vi "ISEG_HVBoardGUI.constructor.vi"(0 "name":string, 2 "data in":string, 5 "error in (no error)":errorcluster) -> (14 "i ref out":refnum<vi>, 16 "data out":string, 19 "error out":errorcluster)   [LabVIEW 2014, in "ISEG_HVBoardGUI.lvlib"]
doc: "This is the constructor of a class.\n\nLicense Agreement for this software:\n\nCopyright (C)\nGesellschaft für Schwerionenforschung, GSI\nPlanckstr. 1\n64291 Darmstadt\nGermany\n\nContact: D.Beck@gsi.de \n\nThis program is free software; you can redistribute it and/or modify it under the terms of the \nGNU General Public License as published by the Free Software Foundation; either version 2 of \nthe license, or (at your option) any later version.\n\nThis program is distributed in the hope that it will be useful, but WITHOUT ANY WARRANTY; \nwithout even the implied warranty of MERCHANTABILITY or FITNESS FOR A PARTICULAR PURPOSE. See the GNU General License for more details (http://www.gnu.org).\n\nGesellschaft für Schwerionenforschung, GSI\nPlanckstr. 1, 64291 Darmstadt, Germany\nFor all questions and ideas contact: M.Richter@gsi.de, H.Brand@gsi.de or D.Beck@gsi.de.\nLast update: 16-JUN-2004"
uses:
  ISEG_HVBoardGUI.lvlib
  ISEG_HVBoardGUI.i attribute.ctl
  CS_Core/CSObj/CSObj.lvlib
  CS_Core/BaseGUI/BaseGUI.lvlib
  CS_Core/CSSystem/CSSystemLib/CSSystemLib.lvlib
panel:
  in  "CLASS.i attribute":T1
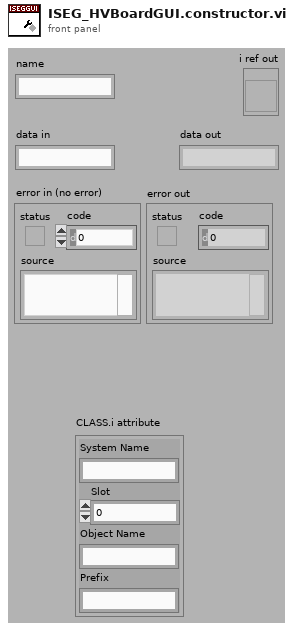
[diagram p1: front panel]
types:
  T1 = typedef "ISEG_HVBoardGUI.lvlib/ISEG_HVBoardGUI.i attribute.ctl" = cluster{"System Name":string, "Slot":i16, "Object Name":string, "Prefix":string}
  T2 = enum16{"SetAttribute", "GetAttribute", "CreateAttribute", "DestroyAttribute", "DestroyAllAtributes"}
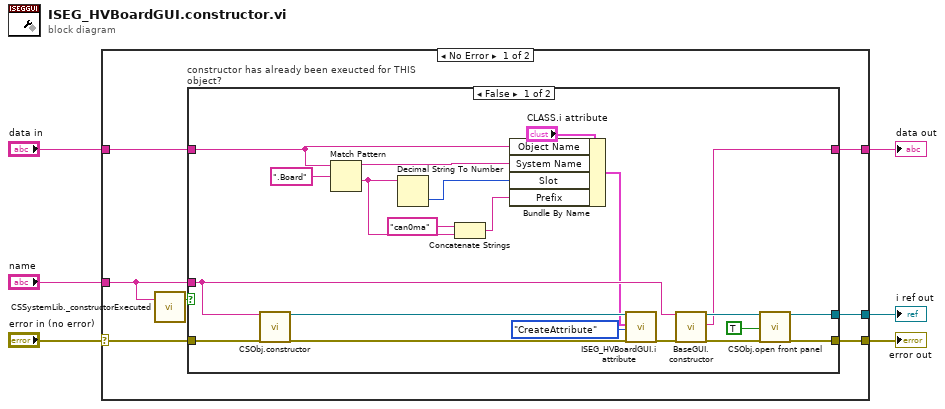
[diagram p0: block diagram]
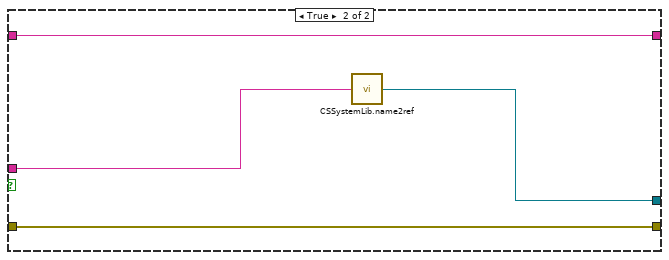
[diagram p2: hidden frame]
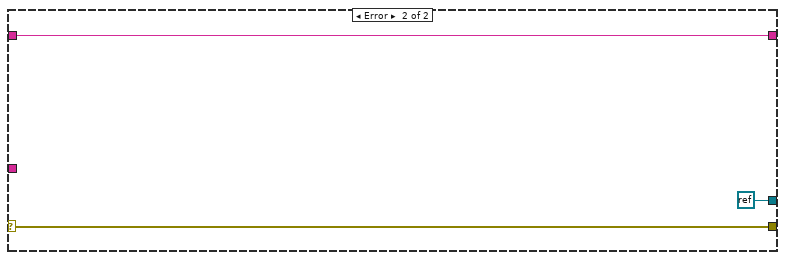
[diagram p3: hidden frame]
diagram:
  n1 = case shown="No Error" "error in (no error)" {
    selector: "error in (no error)" -> [w10 w40]
    tunnel: "data in" -> [w13 w39]
    tunnel: "name" -> [w9 _]
    tunnel: [w12 refnum<k0> refnum] -> w4
    tunnel: [w11 w40] -> w3
    tunnel: [w7 w39] -> w1
    frame No Error {
      n2 = call "CSSystemLib._constructorExecuted.vi"("name"=w9) -> ("constructor executed?"=w8:bool)  [unwired: 18 in]
      n3 = case "constructor has already been exeucted for THIS object?" shown="False" w8 {
        tunnel: w13 -> [w15 w35]
        tunnel: w9 -> [w31 w38]
        tunnel: [w24 w37] -> w12
        tunnel: [w26 w36] -> w11
        tunnel: w10 -> [w29 w36]
        tunnel: [w16 w35] -> w7
        frame False {
          n4 = call "CSObj.constructor.vi"("name"=w31, "error in (no error)"=w29) -> ("i ref out"=w33:refnum<vi>, "error out"=w32:errorcluster)  [unwired: 15 in, 1 out]
          n5 = Match Pattern(string=w15, regular expression=".Board") -> (before substring=w14:string, after substring=w18:string)  [unwired: 1 in, 2 out]
          n6 = Decimal String To Number(string=w18) -> (number=w17:i32)  [unwired: 2 in, 1 out]
          n7 = Concatenate Strings("can0ma", w18) -> (w19:string)
          n8 = Bundle By Name(cluster="CLASS.i attribute", "Object Name"=w15, "System Name"=w14, "Slot"=w17, "Prefix"=w19) -> (w23:T1)
          n9 = call "ISEG_HVBoardGUI.i attribute.vi"("VI Refnum"=w33, "CLASS.i attribute"=w23, "Action"=T2."CreateAttribute", "error in (no error)"=w32) -> ("error out"=w30:errorcluster)  [unwired: 13 in, 2 out]
          n10 = call "BaseGUI.constructor.vi"("name"=w31, "error in (no error)"=w30) -> ("i ref out"=w25:refnum<vi>, "data out"=w16:string, "error out"=w27:errorcluster)  [unwired: 15 in]
          n11 = call "CSObj.open front panel.vi"("i ref in"=w25, "frontPanelOpen"=TRUE ("front panel open"), "error in (no error)"=w27) -> ("i ref out"=w24:refnum<vi>, "error out"=w26:errorcluster)  [unwired: 15 in]
        }
        frame True {
          n12 = call "CSSystemLib.name2ref.vi"("name"=w38) -> ("obj refnum"=w37:refnum<vi>)
        }
      }
    }
    frame Error {
    }
  }
  "i ref out" <- w4
  "error out" <- w3
  "data out" <- w1
